vi "observacao.vi"() -> ()   [LabVIEW 2012] (continued)
                  frame True {
                    w2978 = u16 4 items=["ZERO", "AH", "DEC", "TUBO", "CUP"] ("Controlador")
                    n2288 = call "Monta Comando.vi"("Comando"="SUBIR", "Dispositivo"="PARAVENTO" ("Comando"), "Controlador"=w2978) -> ()  [unwired: 4 in, 3 out]
                  }
                }
              }
              event "BtParavDown": Value Change {
                n2289 = event-data() -> ("NewVal"=w2979:bool)  [unwired: 1 in, 5 out]
                n2290 = case shown="True" w2979 {
                  frame False {
                  }
                  frame True {
                    w2982 = u16 4 items=["ZERO", "AH", "DEC", "TUBO", "CUP"] ("Controlador")
                    n2291 = call "Monta Comando.vi"("Comando"="DESCER", "Dispositivo"="PARAVENTO" ("Comando"), "Controlador"=w2982) -> ()  [unwired: 4 in, 3 out]
                  }
                }
              }
              event "BtParavStop": Value Change {
                n2292 = event-data() -> ("NewVal"=w2983:bool)  [unwired: 1 in, 5 out]
                n2293 = case shown="True" w2983 {
                  frame False {
                  }
                  frame True {
                    w2986 = u16 4 items=["ZERO", "AH", "DEC", "TUBO", "CUP"] ("Controlador")
                    n2294 = call "Monta Comando.vi"("Comando"="PARAR", "Dispositivo"="PARAVENTO" ("Comando"), "Controlador"=w2986) -> ()  [unwired: 4 in, 3 out]
                  }
                }
              }
            }
            n2295 = global read "Global_Telescopio.vi" "PosCUP"() -> (w2830:i16)
            n2296 = local read "RefreshShutterState"() -> (w2831:bool)
            n2297 = call "Bit Status CUP.vi"("NomeStatus"=w2833) -> ("StatBit"=w2832:bool)
            "LedShutter" <- w2832
            n2298 = case shown="\"Stopping\"" w2838 {
              tunnel: w2834 -> [_ w2908 w2915 w2918]
              tunnel: w2835 -> [_ _ _ _]
              frame "", Default {
              }
              frame "Not Ready" {
                n2299 = case shown="False" w2908 {
                  frame False {
                    w2914 = u16 4 items=["ZERO", "AH", "DEC", "TUBO", "CUP"] ("Controlador")
                    n2300 = local read "DestCUP"() -> (w2910:i16)
                    n2301 = local write "StatDome"("Moving" ("Status")) -> ()
                    n2302 = Number To Decimal String(number=w2910) -> (decimal integer string=w2911:string)  [unwired: 1 in]
                    n2303 = call "Monta Comando.vi"("Set Point"=w2911, "Comando"="MOVER", "Dispositivo"="DOMO" ("Comando"), "Controlador"=w2914) -> ()  [unwired: 3 in, 3 out]
                  }
                  frame True {
                  }
                }
              }
              frame "Stopping" {
                n2304 = case shown="False" w2915 {
                  frame False {
                    # "Reabilita Abas"
                    n2305 = property on="Setup, Pointing & Guiding" class="TabCtl (strict)"("Page Selector Visible"=TRUE) -> ()  [unwired: 2 in, 2 out]
                    n2306 = local write "StatDome"("Stopped" ("Status")) -> ()
                  }
                  frame True {
                  }
                }
              }
              frame "Moving" {
                n2307 = case shown="False" w2918 {
                  frame False {
                    # "Reabilita Abas"
                    n2308 = property on="Setup, Pointing & Guiding" class="TabCtl (strict)"("Page Selector Visible"=TRUE) -> ()  [unwired: 2 in, 2 out]
                    n2309 = local write "StatDome"("Stopped" ("Status")) -> ()
                  }
                  frame True {
                  }
                }
              }
            }
            n2310 = case shown="\"Busy to Close\"" w2836 {
              tunnel: w2835 -> [_ _ _ _]
              tunnel: w2834 -> [_ w2891 w2897 _]
              frame "", Default {
              }
              frame "Busy to Open" {
                n2311 = case shown="False" w2891 {
                  frame False {
                    w2895 = u16 4 items=["ZERO", "AH", "DEC", "TUBO", "CUP"] ("Controlador")
                    n2312 = call "TickTimeout.vi"() -> ("msTick"=w2892:u32)  [unwired: 2 in, 2 out]
                    n2313 = local write "TimeoutTrap"(w2892) -> ()
                    n2314 = local write "StatShutter"("Moving" ("Status")) -> ()
                    n2315 = call "Monta Comando.vi"("Comando"="ABRIR", "Dispositivo"="TRAPEIRA" ("Comando"), "Controlador"=w2895) -> ()  [unwired: 4 in, 3 out]
                  }
                  frame True {
                  }
                }
              }
              frame "Busy to Close" {
                n2316 = case shown="False" w2897 {
                  frame False {
                    w2901 = u16 4 items=["ZERO", "AH", "DEC", "TUBO", "CUP"] ("Controlador")
                    n2317 = call "TickTimeout.vi"() -> ("msTick"=w2898:u32)  [unwired: 2 in, 2 out]
                    n2318 = local write "TimeoutTrap"(w2898) -> ()
                    n2319 = local write "StatShutter"("Moving" ("Status")) -> ()
                    n2320 = call "Monta Comando.vi"("Comando"="FECHAR", "Dispositivo"="TRAPEIRA" ("Comando"), "Controlador"=w2901) -> ()  [unwired: 4 in, 3 out]
                  }
                  frame True {
                  }
                }
              }
              frame "Moving" {
                n2321 = local read "TimeoutTrap"() -> (w2903:u32)
                n2322 = call "TickTimeout.vi"("msInicial"=w2903, "msTimeout"=u32 12000) -> ("Timeout"=w2904:bool)  [unwired: 2 out]
                n2323 = case shown="False" w2904 {
                  selector: w2904 -> [w2907 _]
                  frame False {
                    n2324 = Not(x=w2907) -> (.not. x?=w2906:bool)
                    n2325 = local write "RefreshShutterState"(w2906) -> ()
                  }
                  frame True {
                  }
                }
              }
            }
            n2326 = case shown="True" w2831 {
              selector: w2831 -> [_ w2886]
              tunnel: w2832 -> [_ w2887]
              frame False {
              }
              frame True {
                n2327 = Not(x=w2886) -> (.not. x?=→"RefreshShutterState":bool)
                n2328 = Select(t="Opened" ("Status"), s=w2887, f="Closed" ("Status")) -> (s? t:f=w2888:string)
                n2329 = local write "StatShutter"(w2888) -> ()
              }
            }
            n2330 = Divide(x=w2830, y=w2826) -> (x/y=w2841:dbl)
            n2331 = To Word Integer(number=w2841) -> (16bit integer=→"PosCup":i16)
            n2332 = local read "Flag-ShutClose"() -> (w2824:bool)
            n2333 = local read "Flag-ShutOpen"() -> (w2823:bool)
            n2334 = Or(x=w2824, y=w2823) -> (x .or. y?=w2822:bool)
            n2335 = case shown="True" w2822 {
              frame False {
              }
              frame True {
                n2336 = local read "Cont-ShutOpen"() -> (w2863:timestamp)
                n2337 = Get Date/Time In Seconds() -> (seconds since 1Jan1904=w2864:timestamp)
                n2338 = Greater Or Equal?(x=w2864, y=w2863) -> (x >= y?=w2862:bool)
                n2339 = case shown="True" w2862 {
                  frame False {
                  }
                  frame True {
                    w2866 = FALSE ("Flag-ShutClose")
                    # "Reabilita todas Abas"
                    n2340 = local write "Flag-ShutClose"(w2866) -> ()
                    n2341 = local write "Flag-ShutOpen"(w2866) -> ()
                    n2342 = property on="Setup, Pointing & Guiding" class="TabCtl (strict)"("Page Selector Visible"=TRUE) -> ()  [unwired: 2 in, 2 out]
                  }
                }
              }
            }
            n2343 = event shown="[2] \"BtShutOpen\": Value Change" {
              selector: _ -> [_ _ _]
              dyn-events: _ -> [_ _ _]
              timeout: 10 -> [_ _ _]
              event Timeout {
                n2344 = event-data() -> ()  [unwired: 1 in, 2 out]
              }
              event "BtShutClose": Value Change {
                # "Desabilita todas Abas"
                n2345 = event-data() -> ("NewVal"=w2867:bool)  [unwired: 1 in, 4 out]
                n2346 = case shown="True" w2867 {
                  selector: w2867 -> [_ w2872]
                  frame False {
                  }
                  frame True {
                    n2347 = Get Date/Time In Seconds() -> (seconds since 1Jan1904=w2871:timestamp)
                    n2348 = Add(x=w2871, y=10.0) -> (x+y=w2869:timestamp)
                    n2349 = local write "Cont-ShutOpen"(w2869) -> ()
                    n2350 = property on="Setup, Pointing & Guiding" class="TabCtl (strict)"("Page Selector Visible"=FALSE) -> ()  [unwired: 2 in, 2 out]
                    "Flag-ShutClose" <- w2872
                  }
                }
              }
              event "BtShutOpen": Value Change {
                # "Desabilita todas Abas"
                n2351 = event-data() -> ("NewVal"=w2873:bool)  [unwired: 1 in, 4 out]
                n2352 = case shown="True" w2873 {
                  selector: w2873 -> [_ w2874]
                  frame False {
                  }
                  frame True {
                    n2353 = stacked-sequence {
                      tunnel: w2874 -> [w2879 _]
                      frame #0 {
                        n2354 = Get Date/Time In Seconds() -> (seconds since 1Jan1904=w2878:timestamp)
                        n2355 = Add(x=w2878, y=10.0) -> (x+y=→"Cont-ShutOpen":timestamp)
                        n2356 = property on="Setup, Pointing & Guiding" class="TabCtl (strict)"("Page Selector Visible"=FALSE) -> ()  [unwired: 2 in, 2 out]
                        "Flag-ShutOpen" <- w2879
                      }
                      frame #1 {
                        # "Escreve no LOG o estado do shutter"
                        # "Timer para escrever no log\ne enviar comando:\nCUP TRAPEIRA PARAR"
                        n2357 = Tick Count (ms)() -> (millisecond timer value=w2880:u32)
                        n2358 = local write "sendCommandShutter"(TRUE ("writeShutterLog")) -> ()
                        n2359 = local write "timeStatShutterAlert"(w2880) -> ()
                        n2360 = local write "shutterTimeOld"(w2880) -> ()
                        n2361 = call "Log_Shutter.vi"("command"=" ", "domeState"="OPENED " ("command"), "pathLogDomeFile"="C:\\TCS\\LOG\\SHUTTER\\SHUTTER.TXT" ("pathLogFocoString")) -> ()  [unwired: 6 in]
                      }
                    }
                  }
                }
              }
            }
            n2362 = event shown="[3] \"CW\": Mouse Down" {
              selector: _ -> [_ _ _ _ _]
              dyn-events: _ -> [_ _ _ _ _]
              timeout: 100 -> [_ _ _ _ _]
              event Timeout {
                n2363 = event-data() -> ()  [unwired: 1 in, 2 out]
              }
              event "CCW": Mouse Down {
                w2842 = "GIRAR_CCW" ("Comando")
                w2843 = u16 4 items=["ZERO", "AH", "DEC", "TUBO", "CUP"] ("Controlador")
                # "Envia o comando GIRAR"
                n2364 = event-data() -> ()  [unwired: 1 in, 7 out]
                n2365 = local write "Command"(w2842) -> ()
                n2366 = call "Monta Comando.vi"("Comando"=w2842, "Dispositivo"="DOMO" ("Comando"), "Controlador"=w2843) -> ()  [unwired: 4 in, 3 out]
              }
              event "CCW": Mouse Up {
                n2367 = event-data() -> ()  [unwired: 1 in, 7 out]
                n2368 = stacked-sequence {
                  frame #0 {
                    w2845 = "PARAR" ("Comando")
                    w2846 = u16 4 items=["ZERO", "AH", "DEC", "TUBO", "CUP"] ("Controlador")
                    # "Envia o comando PARAR"
                    n2369 = local write "Command"(w2845) -> ()
                    n2370 = call "Monta Comando.vi"("Comando"=w2845, "Dispositivo"="DOMO" ("Comando"), "Controlador"=w2846) -> ()  [unwired: 4 in, 3 out]
                  }
                  frame #1 {
                    n2371 = Wait (ms)(milliseconds to wait=u32 100) -> ()  [unwired: 1 out]
                  }
                  frame #2 {
                    w2849 = "PARAR" ("Comando")
                    w2850 = u16 4 items=["ZERO", "AH", "DEC", "TUBO", "CUP"] ("Controlador")
                    # "Envia o comando PARAR"
                    n2372 = local write "Command"(w2849) -> ()
                    n2373 = call "Monta Comando.vi"("Comando"=w2849, "Dispositivo"="DOMO" ("Comando"), "Controlador"=w2850) -> ()  [unwired: 4 in, 3 out]
                  }
                }
              }
              event "CW": Mouse Down {
                w2852 = "GIRAR_CW" ("Comando")
                w2853 = u16 4 items=["ZERO", "AH", "DEC", "TUBO", "CUP"] ("Controlador")
                # "Envia o comando GIRAR"
                n2374 = event-data() -> ()  [unwired: 1 in, 7 out]
                n2375 = local write "Command"(w2852) -> ()
                n2376 = call "Monta Comando.vi"("Comando"=w2852, "Dispositivo"="DOMO" ("Comando"), "Controlador"=w2853) -> ()  [unwired: 4 in, 3 out]
              }
              event "CW": Mouse Up {
                n2377 = event-data() -> ()  [unwired: 1 in, 7 out]
                n2378 = stacked-sequence {
                  frame #0 {
                    w2855 = "PARAR" ("Comando")
                    w2856 = u16 4 items=["ZERO", "AH", "DEC", "TUBO", "CUP"] ("Controlador")
                    # "Envia o comando PARAR"
                    n2379 = local write "Command"(w2855) -> ()
                    n2380 = call "Monta Comando.vi"("Comando"=w2855, "Dispositivo"="DOMO" ("Comando"), "Controlador"=w2856) -> ()  [unwired: 4 in, 3 out]
                  }
                  frame #1 {
                    n2381 = Wait (ms)(milliseconds to wait=u32 100) -> ()  [unwired: 1 out]
                  }
                  frame #2 {
                    w2859 = "PARAR" ("Comando")
                    w2860 = u16 4 items=["ZERO", "AH", "DEC", "TUBO", "CUP"] ("Controlador")
                    # "Envia o comando PARAR"
                    n2382 = local write "Command"(w2859) -> ()
                    n2383 = call "Monta Comando.vi"("Comando"=w2859, "Dispositivo"="DOMO" ("Comando"), "Controlador"=w2860) -> ()  [unwired: 4 in, 3 out]
                  }
                }
              }
            }
            "Command" <- "" ("Command")
          }
          frame "UTILS " {
            n2384 = stacked-sequence {
              frame #0 {
                # "Acionamento das Abas do\nEspelho\n\nComandos sempre precedidos\nde ESPAÇO\n\nTUBO TAMPAS ESCREVER = 80 80\n\nLigar power geral       08 08\nDesligar power geral  08 00\nLigar System              10 10\nDesligar System         10 00\nPassar para Remoto  20 20\nPassar para Local      20 00\nSel. device central     40 40\nSel. device bowl         40 00\nAction open                80 80\nAction close                80 00"
                n2385 = event shown="[1] \"MODE\": Value Change" {
                  selector: _ -> [_ _ _]
                  dyn-events: _ -> [_ _ _]
                  timeout: 10 -> [_ _ _]
                  event Timeout {
                    n2386 = event-data() -> ()  [unwired: 1 in, 2 out]
                  }
                  event "MODE": Value Change {
                    n2387 = event-data() -> ("NewVal"=w3001:bool)  [unwired: 1 in, 5 out]
                    "LED MODE" <- w3001
                    n2388 = case shown="False" w3001 {
                      frame False {
                        w3006 = u16 3 items=["ZERO", "AH", "DEC", "TUBO", "CUP"] ("Controlador")
                        # "DESABILITA"
                        # "APENAS PASSANDO COMANDO PARA MANETE"
                        # "MODE E GERAL = 0"
                        # "MODE HADSET"
                        n2389 = call "Monta Comando.vi"("Set Point"=" F8 90", "Comando"="ESCREVER", "Dispositivo"="TAMPAS" ("Comando"), "Controlador"=w3006) -> ()  [unwired: 3 in, 3 out]
                        n2390 = property on="ACTION" class="Bool (strict)"("Disabled"=u8 2) -> ()  [unwired: 2 in, 2 out]
                      }
                      frame True {
                        w3011 = u16 3 items=["ZERO", "AH", "DEC", "TUBO", "CUP"] ("Controlador")
                        # "HABILITA"
                        # "APENAS PASSANDO COMOANDO PARA TCSPD"
                        # "MODE E GERAL = 1"
                        # "MODE TCSPD"
                        n2391 = call "Monta Comando.vi"("Set Point"=" 48 48", "Comando"="ESCREVER", "Dispositivo"="TAMPAS" ("Comando"), "Controlador"=w3011) -> ()  [unwired: 3 in, 3 out]
                        n2392 = property on="ACTION" class="Bool (strict)"("Disabled"=u8 0) -> ()  [unwired: 2 in, 2 out]
                      }
                    }
                  }
                  event "ACTION": Value Change {
                    n2393 = event-data() -> ("NewVal"=w3012:bool)  [unwired: 1 in, 5 out]
                    n2394 = case shown="False" w3012 {
                      frame False {
                        # "FECHAR"
                        n2395 = local write "ESTADO FECHAR"("INICIO" ("ESTADO ABRIR")) -> ()
                        n2396 = local write "ESTADO ABRIR"("REPOUSO" ("ESTADO ABRIR")) -> ()
                      }
                      frame True {
                        # "ABRIR"
                        n2397 = local write "ESTADO FECHAR"("REPOUSO" ("ESTADO ABRIR")) -> ()
                        n2398 = local write "ESTADO ABRIR"("INICIO" ("ESTADO ABRIR")) -> ()
                      }
                    }
                  }
                }
                n2399 = Tick Count (ms)() -> (millisecond timer value=w2992:u32)
                n2400 = Greater Or Equal?(x=w2992, y="TIMER TICK") -> (x >= y?=w2988:bool)
                n2401 = And(x=w2988, y=FALSE) -> (x .and. y?=w2989:bool)
                n2402 = case shown="True" w2989 {
                  frame False {
                  }
                  frame True {
                    w3025 = u16 3 items=["ZERO", "AH", "DEC", "TUBO", "CUP", "CASS", "COUDE"] ("Controlador")
                    # "2 SEGUNDOS"
                    n2403 = Tick Count (ms)() -> (millisecond timer value=w3022:u32)
                    n2404 = Add(x=w3022, y=u32 10000) -> (x+y=w3020:u32)
                    n2405 = call "Status_das_Tampas.vi"("Controlador"=w3025, "DISPOSITIVO"="TAMPAS", "Comando"="LER") -> ("Fechado/Aberto"=w3019:bool, "Dispositivo Bacia/Centar"=w3018:bool)  [unwired: 6 in, 5 out]
                    n2406 = local write "TIMER TICK"(w3020) -> ()
                    n2407 = Not(x=w3019) -> (.not. x?=w3017:bool)
                    n2408 = And(x=w3017, y=w3018) -> ()  [unwired: 1 out]
                  }
                }
                n2409 = event shown="[4] \"FLAT-FIELD\": Value Change" {
                  selector: _ -> [_ _ _ _ _ _]
                  dyn-events: _ -> [_ _ _ _ _ _]
                  timeout: 10 -> [_ _ _ _ _ _]
                  event Timeout {
                    n2410 = event-data() -> ()  [unwired: 1 in, 2 out]
                  }
                  event "BtUtilPark": Value Change {
                    n2411 = event-data() -> ("NewVal"=w3026:bool)  [unwired: 1 in, 5 out]
                    n2412 = case shown="True" w3026 {
                      frame False {
                      }
                      frame True {
                        w3029 = u16 4 items=["ZERO", "AH", "DEC", "TUBO", "CUP"] ("Controlador")
                        w3030 = FALSE ("MOUNT")
                        w3033 = 0 ("M_AH")
                        w3034 = u8 2 ("Disabled")
                        w3031 = FALSE ("Page Selector Visible")
                        w3038 = 1 ("M_AH")
                        # "Carrega \nParâmetros \nda Configuração"
                        # "Seta Máq GO"
                        # "Desabilita todas Abas"
                        # "DESABILITA TODOS"
                        n2413 = local write "DOME"(w3031) -> ()
                        n2414 = property on="Setup, Pointing & Guiding" class="TabCtl (strict)"("Page Selector Visible"=w3031) -> ()  [unwired: 2 in, 2 out]
                        n2415 = local write "statAH"(w3033) -> ()
                        n2416 = local write "statCUP"(w3033) -> ()
                        n2417 = local write "statDEC"(w3033) -> ()
                        n2418 = local write "M_DEC"(w3038) -> ()
                        n2419 = local write "M_AH"(w3038) -> ()
                        n2420 = local write "M_CUP"(w3038) -> ()
                        n2421 = global read "Global_Telescopio.vi" "DestDEC"() -> (w3036:dbl)
                        n2422 = global read "Global_Telescopio.vi" "DestCUP"() -> (w3035:i32)
                        n2423 = global read "Global_Telescopio.vi" "DestAH"() -> (w3037:dbl)
                        n2424 = property on="BtUtilPark" class="Bool (strict)"("Disabled"=w3034) -> ()  [unwired: 2 in, 2 out]
                        n2425 = property on="ECASS" class="Bool (strict)"("Disabled"=w3034) -> ()  [unwired: 2 in, 2 out]
                        n2426 = local write "DestAH"(w3037) -> ()
                        n2427 = local write "DestCUP"(w3035) -> ()
                        n2428 = local write "DestDEC"(w3036) -> ()
                        n2429 = global write "Global_Telescopio.vi" "Parking"(TRUE ("Page Selector Visible")) -> ()
                        n2430 = property on="BtUtilZenith" class="Bool (strict)"("Disabled"=w3034) -> ()  [unwired: 2 in, 2 out]
                        n2431 = property on="FLAT-FIELD" class="Bool (strict)"("Disabled"=w3034) -> ()  [unwired: 2 in, 2 out]
                        n2432 = call "Monta Comando.vi"("Comando"="LIGAR", "Dispositivo"="LAMP_CAM" ("Comando"), "Controlador"=w3029) -> ()  [unwired: 4 in, 3 out]
                        n2433 = property on="PROTEÇÃO" class="Bool (strict)"("Disabled"=w3034) -> ()  [unwired: 2 in, 2 out]
                        n2434 = local write "MOUNT"(w3030) -> ()
                        n2435 = local write "GUIDER"(w3030) -> ()
                      }
                    }
                  }
                  event "BtUtilZenith": Value Change {
                    n2436 = event-data() -> ("NewVal"=w3039:bool)  [unwired: 1 in, 5 out]
                    n2437 = case shown="True" w3039 {
                      frame False {
                      }
                      frame True {
                        w3042 = u16 4 items=["ZERO", "AH", "DEC", "TUBO", "CUP"] ("Controlador")
                        w3043 = FALSE ("MOUNT")
                        w3046 = 0 ("M_AH")
                        w3047 = u8 2 ("Disabled")
                        w3045 = FALSE ("Page Selector Visible")
                        w3051 = 1 ("M_AH")
                        # "Seta Máq GO"
                        # "Desabilita todas Abas"
                        # "DESABILITA TODOS"
                        n2438 = local write "M_DEC"(w3051) -> ()
                        n2439 = local write "M_AH"(w3051) -> ()
                        n2440 = local write "M_CUP"(w3051) -> ()
                        n2441 = local write "DOME"(w3045) -> ()
                        n2442 = property on="Setup, Pointing & Guiding" class="TabCtl (strict)"("Page Selector Visible"=w3045) -> ()  [unwired: 2 in, 2 out]
                        n2443 = local write "statAH"(w3046) -> ()
                        n2444 = local write "statCUP"(w3046) -> ()
                        n2445 = local write "statDEC"(w3046) -> ()
                        n2446 = global read "Global_Telescopio.vi" "Telescopio"() -> (w3044:bool)
                        n2447 = property on="BtUtilPark" class="Bool (strict)"("Disabled"=w3047) -> ()  [unwired: 2 in, 2 out]
                        n2448 = property on="ECASS" class="Bool (strict)"("Disabled"=w3047) -> ()  [unwired: 2 in, 2 out]
                        n2449 = case shown="False" w3044 {
                          tunnel: [0.0 ("DestAH") 0.0 ("DestAH")] -> w3050
                          tunnel: [-0.3933 ("DestDEC") -0.3933 ("DestDEC")] -> w3049
                          tunnel: [i16 98 ("DestCUP") i16 80 ("DestCUP")] -> w3048
                          frame False {
                          }
                          frame True {
                          }
                        }
                        n2450 = property on="BtUtilZenith" class="Bool (strict)"("Disabled"=w3047) -> ()  [unwired: 2 in, 2 out]
                        n2451 = property on="FLAT-FIELD" class="Bool (strict)"("Disabled"=w3047) -> ()  [unwired: 2 in, 2 out]
                        n2452 = call "Monta Comando.vi"("Comando"="LIGAR", "Dispositivo"="LAMP_CAM" ("Comando"), "Controlador"=w3042) -> ()  [unwired: 4 in, 3 out]
                        n2453 = local write "DestAH"(w3050) -> ()
                        n2454 = local write "DestCUP"(w3048) -> ()
                        n2455 = local write "DestDEC"(w3049) -> ()
                        n2456 = property on="PROTEÇÃO" class="Bool (strict)"("Disabled"=w3047) -> ()  [unwired: 2 in, 2 out]
                        n2457 = local write "MOUNT"(w3043) -> ()
                        n2458 = local write "GUIDER"(w3043) -> ()
                      }
                    }
                  }
                  event "ECASS": Value Change {
                    n2459 = event-data() -> ("NewVal"=w3058:bool)  [unwired: 1 in, 5 out]
                    n2460 = case shown="True" w3058 {
                      frame False {
                      }
                      frame True {
                        w3061 = u16 4 items=["ZERO", "AH", "DEC", "TUBO", "CUP"] ("Controlador")
                        w3062 = FALSE ("MOUNT")
                        w3065 = 0 ("M_AH")
                        w3066 = u8 2 ("Disabled")
                        w3064 = FALSE ("Page Selector Visible")
                        w3070 = 1 ("M_AH")
                        # "Seta Máq GO"
                        # "Desabilita todas Abas"
                        # "DESABILITA TODOS"
                        n2461 = local write "M_DEC"(w3070) -> ()
                        n2462 = local write "M_AH"(w3070) -> ()
                        n2463 = local write "M_CUP"(w3070) -> ()
                        n2464 = local write "DOME"(w3064) -> ()
                        n2465 = property on="Setup, Pointing & Guiding" class="TabCtl (strict)"("Page Selector Visible"=w3064) -> ()  [unwired: 2 in, 2 out]
                        n2466 = local write "statAH"(w3065) -> ()
                        n2467 = local write "statCUP"(w3065) -> ()
                        n2468 = local write "statDEC"(w3065) -> ()
                        n2469 = global read "Global_Telescopio.vi" "Telescopio"() -> (w3063:bool)
                        n2470 = property on="BtUtilPark" class="Bool (strict)"("Disabled"=w3066) -> ()  [unwired: 2 in, 2 out]
                        n2471 = property on="ECASS" class="Bool (strict)"("Disabled"=w3066) -> ()  [unwired: 2 in, 2 out]
                        n2472 = case shown="False" w3063 {
                          tunnel: [0.0 ("DestAH") 0.0 ("DestAH")] -> w3069
                          tunnel: [0.4 ("DestDEC") 0.4 ("DestDEC")] -> w3068
                          tunnel: [i16 98 ("DestCUP") i16 80 ("DestCUP")] -> w3067
                          frame False {
                          }
                          frame True {
                          }
                        }
                        n2473 = property on="BtUtilZenith" class="Bool (strict)"("Disabled"=w3066) -> ()  [unwired: 2 in, 2 out]
                        n2474 = property on="FLAT-FIELD" class="Bool (strict)"("Disabled"=w3066) -> ()  [unwired: 2 in, 2 out]
                        n2475 = local write "DestAH"(w3069) -> ()
                        n2476 = local write "DestCUP"(w3067) -> ()
                        n2477 = local write "DestDEC"(w3068) -> ()
                        n2478 = call "Monta Comando.vi"("Comando"="LIGAR", "Dispositivo"="LAMP_CAM" ("Comando"), "Controlador"=w3061) -> ()  [unwired: 4 in, 3 out]
                        n2479 = property on="PROTEÇÃO" class="Bool (strict)"("Disabled"=w3066) -> ()  [unwired: 2 in, 2 out]
                        n2480 = local write "GUIDER"(w3062) -> ()
                        n2481 = local write "MOUNT"(w3062) -> ()
                      }
                    }
                  }
                  event "FLAT-FIELD": Value Change {
                    n2482 = event-data() -> ("NewVal"=w3077:bool)  [unwired: 1 in, 5 out]
                    n2483 = case shown="True" w3077 {
                      frame False {
                      }
                      frame True {
                        w3080 = u16 4 items=["ZERO", "AH", "DEC", "TUBO", "CUP"] ("Controlador")
                        w3081 = FALSE ("MOUNT")
                        w3083 = 0 ("M_AH")
                        w3085 = u8 2 ("Disabled")
                        w3084 = FALSE ("Page Selector Visible")
                        w3089 = 1 ("M_AH")
                        # "Seta Máq GO"
                        # "Desabilita todas Abas"
                        # "DESABILITA TODOS"
                        n2484 = local write "M_DEC"(w3089) -> ()
                        n2485 = local write "M_AH"(w3089) -> ()
                        n2486 = local write "M_CUP"(w3089) -> ()
                        n2487 = local write "DOME"(w3084) -> ()
                        n2488 = property on="Setup, Pointing & Guiding" class="TabCtl (strict)"("Page Selector Visible"=w3084) -> ()  [unwired: 2 in, 2 out]
                        n2489 = local write "statAH"(w3083) -> ()
                        n2490 = local write "statCUP"(w3083) -> ()
                        n2491 = local write "statDEC"(w3083) -> ()
                        n2492 = global read "Global_Telescopio.vi" "Telescopio"() -> (w3082:bool)
                        n2493 = property on="BtUtilPark" class="Bool (strict)"("Disabled"=w3085) -> ()  [unwired: 2 in, 2 out]
                        n2494 = property on="ECASS" class="Bool (strict)"("Disabled"=w3085) -> ()  [unwired: 2 in, 2 out]
                        n2495 = case shown="False" w3082 {
                          tunnel: [0.0715 ("DestAH") 0.31416 ("DestAH")] -> w3088
                          tunnel: [0.641 ("DestDEC") -0.39415 ("DestDEC")] -> w3087
                          tunnel: [i16 306 ("DestCUP") i16 133 ("DestCUP")] -> w3086
                          frame False {
                          }
                          frame True {
                          }
                        }
                        n2496 = property on="BtUtilZenith" class="Bool (strict)"("Disabled"=w3085) -> ()  [unwired: 2 in, 2 out]
                        n2497 = property on="FLAT-FIELD" class="Bool (strict)"("Disabled"=w3085) -> ()  [unwired: 2 in, 2 out]
                        n2498 = local write "DestAH"(w3088) -> ()
                        n2499 = local write "DestCUP"(w3086) -> ()
                        n2500 = local write "DestDEC"(w3087) -> ()
                        n2501 = call "Monta Comando.vi"("Comando"="LIGAR", "Dispositivo"="LAMP_CAM" ("Comando"), "Controlador"=w3080) -> ()  [unwired: 4 in, 3 out]
                        n2502 = property on="PROTEÇÃO" class="Bool (strict)"("Disabled"=w3085) -> ()  [unwired: 2 in, 2 out]
                        n2503 = local write "GUIDER"(w3081) -> ()
                        n2504 = local write "MOUNT"(w3081) -> ()
                      }
                    }
                  }
                  event "PROTEÇÃO": Value Change {
                    n2505 = event-data() -> ("NewVal"=w3096:bool)  [unwired: 1 in, 5 out]
                    n2506 = case shown="True" w3096 {
                      frame False {
                      }
                      frame True {
                        w3097 = FALSE ("MOUNT")
                        w3099 = 0 ("M_AH")
                        w3098 = FALSE ("Page Selector Visible")
                        w3101 = u8 2 ("Disabled")
                        # "Seta Máq GO"
                        # "Desabilita todas Abas"
                        # "DESABILITA TODOS"
                        n2507 = local write "DOME"(w3098) -> ()
                        n2508 = property on="Setup, Pointing & Guiding" class="TabCtl (strict)"("Page Selector Visible"=w3098) -> ()  [unwired: 2 in, 2 out]
                        n2509 = local write "statAH"(w3099) -> ()
                        n2510 = local write "statCUP"(w3099) -> ()
                        n2511 = local write "statDEC"(w3099) -> ()
                        n2512 = property on="BtUtilPark" class="Bool (strict)"("Disabled"=w3101) -> ()  [unwired: 2 in, 2 out]
                        n2513 = property on="ECASS" class="Bool (strict)"("Disabled"=w3101) -> ()  [unwired: 2 in, 2 out]
                        n2514 = property on="BtUtilZenith" class="Bool (strict)"("Disabled"=w3101) -> ()  [unwired: 2 in, 2 out]
                        n2515 = property on="FLAT-FIELD" class="Bool (strict)"("Disabled"=w3101) -> ()  [unwired: 2 in, 2 out]
                        n2516 = local write "M_PROT"(1 ("M_PROT")) -> ()
                        n2517 = local write "GUIDER"(w3097) -> ()
                        n2518 = local write "MOUNT"(w3097) -> ()
                        n2519 = property on="PROTEÇÃO" class="Bool (strict)"("Disabled"=w3101) -> ()  [unwired: 2 in, 2 out]
                      }
                    }
                  }
                }
                n2520 = case shown="True" "STOP" {
                  frame False {
                  }
                  frame True {
                    n2521 = stacked-sequence {
                      frame #0 {
                        w3103 = 0 ("estado")
                        # "Zera Máquina de Estado\nPelo Botão STOP"
                        n2522 = property on="Setup, Pointing & Guiding" class="TabCtl (strict)"("Page Selector Visible"=TRUE) -> ()  [unwired: 2 in, 2 out]
                        n2523 = call "Stop.vi"() -> ()  [unwired: 1 in, 1 out]
                        n2524 = local write "Flag Stop"(TRUE ("Flag Stop")) -> ()
                        n2525 = local write "M_AH"(w3103) -> ()
                        n2526 = local write "M_DEC"(w3103) -> ()
                        n2527 = local write "M_CUP"(w3103) -> ()
                        n2528 = local write "M_PROT"(w3103) -> ()
                      }
                      frame #1 {
                        w3105 = FALSE
                        w3106 = u8 0 ("Disabled")
                        # "DESLIGA TODOS"
                        # "HABILITA TODOS"
                        n2529 = local write "BtUtilZenith"(w3105) -> ()
                        n2530 = local write "BtUtilPark"(w3105) -> ()
                        n2531 = local write "FLAT-FIELD"(w3105) -> ()
                        n2532 = local write "PROTEÇÃO"(w3105) -> ()
                        n2533 = local write "ECASS"(w3105) -> ()
                        n2534 = property on="BtUtilPark" class="Bool (strict)"("Disabled"=w3106) -> ()  [unwired: 2 in, 2 out]
                        n2535 = property on="ECASS" class="Bool (strict)"("Disabled"=w3106) -> ()  [unwired: 2 in, 2 out]
                        n2536 = property on="BtUtilZenith" class="Bool (strict)"("Disabled"=w3106) -> ()  [unwired: 2 in, 2 out]
                        n2537 = property on="PROTEÇÃO" class="Bool (strict)"("Disabled"=w3106) -> ()  [unwired: 2 in, 2 out]
                        n2538 = property on="FLAT-FIELD" class="Bool (strict)"("Disabled"=w3106) -> ()  [unwired: 2 in, 2 out]
                      }
                    }
                  }
                }
                n2539 = Compound Arithmetic op=OR("BtUtilPark", "BtUtilZenith", "ECASS", "FLAT-FIELD", "PROTEÇÃO") -> (→"MOVING":bool)
              }
              frame #1 {
                # "MÁQUINAS DE ESTADOS DAS TAMPAS"
                n2540 = case shown="False" "Case Constant\n(See Context Help) 11" {
                  frame False {
                    # "ABRIR"
                    # "FECHAR"
                    n2541 = case shown="\"PIZZA\"" "ESTADO FECHAR" {
                      tunnel: [w3157 w3165 w3176 w3184 w3194 w3202 w3212 "REPOUSO" ("y")] -> w3111
                      frame "INICIO", Default {
                        w3162 = u16 3 items=["ZERO", "AH", "DEC", "TUBO", "CUP"] ("Controlador")
                        # "SELECIONA DISPOSITVO BACIA E\nMANDA FECHAR"
                        # "DISP=1 E PIZZA=1"
                        n2542 = call "Monta Comando.vi"("Set Point"=" A0 A0", "Comando"="ESCREVER", "Dispositivo"="TAMPAS" ("Comando"), "Controlador"=w3162) -> ("Resposta"=w3158:string)  [unwired: 3 in, 2 out]
                        n2543 = Not Equal?(x=w3158, y="TAMPAS OK") -> ()  [unwired: 1 out]
                        n2544 = Tick Count (ms)() -> (millisecond timer value=→"T1 2":u32)
                        n2545 = Select(t="REPOUSO" ("y"), s=FALSE, f="ESPERA 1" ("y")) -> (s? t:f=w3157:string)
                      }
                      frame "ESPERA 1" {
                        # "20 SEGUNDOS"
                        n2546 = local read "T1 2"() -> (w3170:u32)
                        n2547 = Tick Count (ms)() -> (millisecond timer value=w3168:u32)
                        n2548 = Add(x=w3170, y=u32 20000) -> (x+y=w3167:u32)
                        n2549 = Greater?(x=w3168, y=w3167) -> (0:w3164:bool)
                        n2550 = Select(t="PIZZA" ("y"), s=w3164, f="ESPERA 1" ("y")) -> (s? t:f=w3165:string)
                      }
                      frame "PIZZA" {
                        w3181 = u16 3 items=["ZERO", "AH", "DEC", "TUBO", "CUP"] ("Controlador")
                        # "SELECIONA DISP PIZZA\nE MANDA FECHAR"
                        # "PIZZA=1"
                        n2551 = call "Monta Comando.vi"("Set Point"=" 30 10", "Comando"="ESCREVER", "Dispositivo"="TAMPAS" ("Comando"), "Controlador"=w3181) -> ("Resposta"=w3175:string)  [unwired: 3 in, 2 out]
                        n2552 = Tick Count (ms)() -> (millisecond timer value=→"T2 2":u32)
                        n2553 = Not Equal?(x=w3175, y="TAMPAS OK") -> ()  [unwired: 1 out]
                        n2554 = Select(t="REPOUSO" ("y"), s=FALSE, f="PIZZA 2") -> (s? t:f=w3176:string)
                      }
                      frame "PIZZA 2" {
                        w3192 = u16 3 items=["ZERO", "AH", "DEC", "TUBO", "CUP"] ("Controlador")
                        n2555 = call "Monta Comando.vi"("Set Point"=" F8 90", "Comando"="ESCREVER", "Dispositivo"="TAMPAS" ("Comando"), "Controlador"=w3192) -> ("Resposta"=w3187:string)  [unwired: 3 in, 2 out]
                        n2556 = Tick Count (ms)() -> (millisecond timer value=→"T2 3":u32)
                        n2557 = Not Equal?(x=w3187, y="TAMPAS OK") -> ()  [unwired: 1 out]
                        n2558 = Select(t="REPOUSO" ("y"), s=FALSE, f="ESPERA 1A") -> (s? t:f=w3184:string)
                      }
                      frame "ESPERA 1A" {
                        # "2 SEGUNDOS"
                        n2559 = local read "T2 3"() -> (w3197:u32)
                        n2560 = Tick Count (ms)() -> (millisecond timer value=w3199:u32)
                        n2561 = Add(x=w3197, y=u32 2000) -> (x+y=w3200:u32)
                        n2562 = Greater?(x=w3199, y=w3200) -> (0:w3193:bool)
                        n2563 = Select(t="PIZZA 3" ("y"), s=w3193, f="ESPERA 1A" ("y")) -> (s? t:f=w3194:string)
                      }
                      frame "PIZZA 3" {
                        w3210 = u16 3 items=["ZERO", "AH", "DEC", "TUBO", "CUP"] ("Controlador")
                        # "PIZZA=3"
                        n2564 = call "Monta Comando.vi"("Set Point"=" 48 48", "Comando"="ESCREVER", "Dispositivo"="TAMPAS" ("Comando"), "Controlador"=w3210) -> ("Resposta"=w3205:string)  [unwired: 3 in, 2 out]
                        n2565 = Not Equal?(x=w3205, y="TAMPAS OK") -> ()  [unwired: 1 out]
                        n2566 = Select(t="REPOUSO" ("y"), s=FALSE, f="ESPERA 2" ("y")) -> (s? t:f=w3202:string)
                      }
                      frame "ESPERA 2" {
                        # "10 SEGUNDOS"
                        n2567 = local read "T2 2"() -> (w3216:u32)
                        n2568 = Tick Count (ms)() -> (millisecond timer value=w3214:u32)
                        n2569 = Add(x=w3216, y=u32 10000) -> (x+y=w3213:u32)
                        n2570 = Greater?(x=w3214, y=w3213) -> (0:w3211:bool)
                        n2571 = case shown="True" w3211 {
                          frame False {
                          }
                          frame True {
                            n2572 = local write "LED ACTION"(FALSE ("LED ACTION")) -> ()
                          }
                        }
                        n2573 = Select(t="REPOUSO" ("y"), s=w3211, f="ESPERA 2" ("y")) -> (s? t:f=w3212:string)
                      }
                      frame "REPOUSO" {
                      }
                    }
                    n2574 = local write "ESTADO FECHAR"(w3111) -> ()
                    n2575 = case shown="\"INICIO\", Default" "ESTADO ABRIR" {
                      tunnel: [w3116 w3125 w3136 w3143 "REPOUSO" ("y")] -> w3109
                      frame "INICIO", Default {
                        w3122 = u16 3 items=["ZERO", "AH", "DEC", "TUBO", "CUP"] ("Controlador")
                        # "SELECIONA DISPOSITVO PIZZA E\nMANDA ABRIR"
                        # "DISP=0 E PIZZA=0"
                        n2576 = call "Monta Comando.vi"("Set Point"=" 30 00", "Comando"="ESCREVER", "Dispositivo"="TAMPAS" ("Comando"), "Controlador"=w3122) -> ("Resposta"=w3117:string)  [unwired: 3 in, 2 out]
                        n2577 = Not Equal?(x=w3117, y="TAMPAS OK") -> ()  [unwired: 1 out]
                        n2578 = Tick Count (ms)() -> (millisecond timer value=→"T1":u32)
                        n2579 = Select(t="REPOUSO" ("y"), s=FALSE, f="ESPERA 1" ("y")) -> (s? t:f=w3116:string)
                      }
                      frame "ESPERA 1" {
                        # "10 SEGUNDOS"
                        n2580 = local read "T1"() -> (w3130:u32)
                        n2581 = Tick Count (ms)() -> (millisecond timer value=w3128:u32)
                        n2582 = Add(x=w3130, y=u32 10000) -> (x+y=w3127:u32)
                        n2583 = Greater?(x=w3128, y=w3127) -> (0:w3124:bool)
                        n2584 = Select(t="BACIA" ("y"), s=w3124, f="ESPERA 1" ("y")) -> (s? t:f=w3125:string)
                      }
                      frame "BACIA" {
                        w3141 = u16 3 items=["ZERO", "AH", "DEC", "TUBO", "CUP"] ("Controlador")
                        # "SELECIONA DISP BACIA\nE MANDA ABRIR"
                        # "BACIA=0"
                        n2585 = call "Monta Comando.vi"("Set Point"=" A0 20", "Comando"="ESCREVER", "Dispositivo"="TAMPAS" ("Comando"), "Controlador"=w3141) -> ("Resposta"=w3135:string)  [unwired: 3 in, 2 out]
                        n2586 = Tick Count (ms)() -> (millisecond timer value=→"T2":u32)
                        n2587 = Not Equal?(x=w3135, y="TAMPAS OK") -> ()  [unwired: 1 out]
                        n2588 = Select(t="REPOUSO" ("y"), s=FALSE, f="ESPERA 2") -> (s? t:f=w3136:string)
                      }
                      frame "ESPERA 2" {
                        # "25 SEGUNDOS"
                        n2589 = local read "T2"() -> (w3147:u32)
                        n2590 = Tick Count (ms)() -> (millisecond timer value=w3145:u32)
                        n2591 = Add(x=w3147, y=u32 25000) -> (x+y=w3144:u32)
                        n2592 = Greater?(x=w3145, y=w3144) -> (0:w3142:bool)
                        n2593 = case shown="True" w3142 {
                          frame False {
                          }
                          frame True {
                            n2594 = local write "LED ACTION"(TRUE ("LED ACTION")) -> ()
                          }
                        }
                        n2595 = Select(t="REPOUSO" ("y"), s=w3142, f="ESPERA 2" ("y")) -> (s? t:f=w3143:string)
                      }
                      frame "REPOUSO" {
                      }
                    }
                    n2596 = local write "ESTADO ABRIR"(w3109) -> ()
                  }
                  frame True {
                    # "NOVO"
                    # "ABRIR"
                    # "FECHAR"
                    n2597 = local read "ESTADO FECHAR"() -> (w3224:string)
                    n2598 = case shown="\"INICIO\", Default" w3224 {
                      tunnel: [w3289 w3297 w3308 w3316 w3324 "REPOUSO" ("y")] -> w3223
                      frame "INICIO", Default {
                        w3294 = u16 3 items=["ZERO", "AH", "DEC", "TUBO", "CUP"] ("Controlador")
                        # "SELECIONA DISPOSITVO BACIA E\nMANDA FECHAR"
                        n2599 = call "Monta Comando.vi"("Set Point"=" A0 A0", "Comando"="ESCREVER", "Dispositivo"="TAMPAS" ("Comando"), "Controlador"=w3294) -> ("Resposta"=w3290:string)  [unwired: 3 in, 2 out]
                        n2600 = Not Equal?(x=w3290, y="TAMPAS OK") -> ()  [unwired: 1 out]
                        n2601 = Tick Count (ms)() -> (millisecond timer value=→"TF1":u32)
                        n2602 = Select(t="REPOUSO" ("y"), s=FALSE, f="ESPERA1" ("y")) -> (s? t:f=w3289:string)
                      }
                      frame "ESPERA1" {
                        # "20 SEGUNDOS"
                        n2603 = local read "TF1"() -> (w3302:u32)
                        n2604 = Tick Count (ms)() -> (millisecond timer value=w3300:u32)
                        n2605 = Add(x=w3302, y=u32 20000) -> (x+y=w3299:u32)
                        n2606 = Greater?(x=w3300, y=w3299) -> (0:w3296:bool)
                        n2607 = Select(t="PIZZA" ("y"), s=w3296, f="ESPERA1" ("y")) -> (s? t:f=w3297:string)
                      }
                      frame "PIZZA" {
                        w3313 = u16 3 items=["ZERO", "AH", "DEC", "TUBO", "CUP"] ("Controlador")
                        # "PASSA PARA MODO\nHANDSET E PIZZA FECHA"
                        n2608 = call "Monta Comando.vi"("Set Point"=" 48 00", "Comando"="ESCREVER", "Dispositivo"="TAMPAS" ("Comando"), "Controlador"=w3313) -> ("Resposta"=w3307:string)  [unwired: 3 in, 2 out]
                        n2609 = Tick Count (ms)() -> (millisecond timer value=→"TF2":u32)
                        n2610 = Not Equal?(x=w3307, y="TAMPAS OK") -> ()  [unwired: 1 out]
                        n2611 = Select(t="REPOUSO" ("y"), s=FALSE, f="ESPERA2") -> (s? t:f=w3308:string)
                      }
                      frame "ESPERA2" {
                        # "10 SEGUNDOS"
                        n2612 = local read "TF2"() -> (w3314:u32)
                        n2613 = Tick Count (ms)() -> (millisecond timer value=w3320:u32)
                        n2614 = Add(x=w3314, y=u32 10000) -> (x+y=w3321:u32)
                        n2615 = Greater?(x=w3320, y=w3321) -> (0:w3315:bool)
                        n2616 = Select(t="PIZZA3" ("y"), s=w3315, f="ESPERA2" ("y")) -> (s? t:f=w3316:string)
                      }
                      frame "PIZZA3" {
                        w3332 = u16 3 items=["ZERO", "AH", "DEC", "TUBO", "CUP"] ("Controlador")
                        n2617 = case shown="True" "Case Constant\n(See Context Help) 12" {
                          frame False {
                          }
                          frame True {
                            n2618 = local write "LED ACTION"(FALSE ("LED ACTION")) -> ()
                          }
                        }
                        n2619 = call "Monta Comando.vi"("Set Point"=" 48 48", "Comando"="ESCREVER", "Dispositivo"="TAMPAS" ("Comando"), "Controlador"=w3332) -> ("Resposta"=w3327:string)  [unwired: 3 in, 2 out]
                        n2620 = Not Equal?(x=w3327, y="TAMPAS OK") -> ()  [unwired: 1 out]
                        n2621 = Select(t="REPOUSO" ("y"), s=FALSE, f="REPOUSO" ("y")) -> (s? t:f=w3324:string)
                      }
                      frame "REPOUSO" {
                      }
                    }
                    n2622 = local write "ESTADO FECHAR"(w3223) -> ()
                    n2623 = local read "ESTADO ABRIR"() -> (w3222:string)
                    n2624 = case shown="\"INICIO\", Default" w3222 {
                      tunnel: [w3229 w3237 w3245 w3255 w3264 w3277 "REPOUSO" ("y")] -> w3221
                      frame "INICIO", Default {
                        w3235 = u16 3 items=["ZERO", "AH", "DEC", "TUBO", "CUP"] ("Controlador")
                        # "PASSA PARA MODO HANDSET"
                        n2625 = call "Monta Comando.vi"("Set Point"=" F8 00", "Comando"="ESCREVER", "Dispositivo"="TAMPAS" ("Comando"), "Controlador"=w3235) -> ("Resposta"=w3230:string)  [unwired: 3 in, 2 out]
                        n2626 = Not Equal?(x=w3230, y="TAMPAS OK") -> ()  [unwired: 1 out]
                        n2627 = Tick Count (ms)() -> (millisecond timer value=→"TA1":u32)
                        n2628 = Select(t="REPOUSO" ("y"), s=FALSE, f="ESPERA1" ("y")) -> (s? t:f=w3229:string)
                      }
                      frame "ESPERA1" {
                        # "1 SEGUNDO"
                        n2629 = local read "TA1"() -> (w3236:u32)
                        n2630 = Tick Count (ms)() -> (millisecond timer value=w3242:u32)
                        n2631 = Add(x=w3236, y=u32 1000) -> (x+y=w3241:u32)
                        n2632 = Greater?(x=w3242, y=w3241) -> (0:w3239:bool)
                        n2633 = Select(t="ABREPIZZA" ("y"), s=w3239, f="ESPERA1" ("y")) -> (s? t:f=w3237:string)
                      }
                      frame "ABREPIZZA" {
                        w3254 = u16 3 items=["ZERO", "AH", "DEC", "TUBO", "CUP"] ("Controlador")
                        # "MANDA PIZZA ABRIR"
                        n2634 = call "Monta Comando.vi"("Set Point"=" 48 48", "Comando"="ESCREVER", "Dispositivo"="TAMPAS" ("Comando"), "Controlador"=w3254) -> ("Resposta"=w3249:string)  [unwired: 3 in, 2 out]
                        n2635 = Not Equal?(x=w3249, y="TAMPAS OK") -> ()  [unwired: 1 out]
                        n2636 = Tick Count (ms)() -> (millisecond timer value=→"TA2":u32)
                        n2637 = Select(t="ABREPIZZA" ("y"), s=FALSE, f="ESPERA2" ("y")) -> (s? t:f=w3245:string)
                      }
                      frame "ESPERA2" {
                        # "10 SEGUNDOS"
                        n2638 = local read "TA2"() -> (w3256:u32)
                        n2639 = Tick Count (ms)() -> (millisecond timer value=w3261:u32)
                        n2640 = Add(x=w3256, y=u32 10000) -> (x+y=w3260:u32)
                        n2641 = Greater?(x=w3261, y=w3260) -> (0:w3258:bool)
                        n2642 = Select(t="BACIAABRINDO" ("y"), s=w3258, f="ESPERA2" ("y")) -> (s? t:f=w3255:string)
                      }
                      frame "BACIAABRINDO" {
                        w3273 = u16 3 items=["ZERO", "AH", "DEC", "TUBO", "CUP"] ("Controlador")
                        # "BACIA ABRINDO"
                        n2643 = call "Monta Comando.vi"("Set Point"=" A0 20", "Comando"="ESCREVER", "Dispositivo"="TAMPAS" ("Comando"), "Controlador"=w3273) -> ("Resposta"=w3268:string)  [unwired: 3 in, 2 out]
                        n2644 = Not Equal?(x=w3268, y="TAMPAS OK") -> ()  [unwired: 1 out]
                        n2645 = Tick Count (ms)() -> (millisecond timer value=→"TA3":u32)
                        n2646 = Select(t="BACIAABRINDO" ("y"), s=FALSE, f="ESPERA3" ("y")) -> (s? t:f=w3264:string)
                      }
                      frame "ESPERA3" {
                        # "25 SEGUNDOS"
                        n2647 = local read "TA3"() -> (w3275:u32)
                        n2648 = Tick Count (ms)() -> (millisecond timer value=w3280:u32)
                        n2649 = Add(x=w3275, y=u32 25000) -> (x+y=w3279:u32)
                        n2650 = Greater?(x=w3280, y=w3279) -> (0:w3274:bool)
                        n2651 = case shown="True" w3274 {
                          frame False {
                          }
                          frame True {
                            n2652 = local write "LED ACTION"(TRUE ("LED ACTION")) -> ()
                          }
                        }
                        n2653 = Select(t="REPOUSO" ("y"), s=w3274, f="ESPERA3" ("y")) -> (s? t:f=w3277:string)
                      }
                      frame "REPOUSO" {
                      }
                    }
                    n2654 = local write "ESTADO ABRIR"(w3221) -> ()
                  }
                }
              }
              frame #2 {
                # "MÁQUINA DE ESTADOS PROTEÇÃO"
                n2655 = case shown="3" "M_PROT" {
                  selector: "M_PROT" -> [w3338 _ _ _ _ _]
                  tunnel: [w3338 w3339 w3358 5 5 ("estadoCUP") 0 ("estadoCUP")] -> w3336
                  frame 0, Default {
                    # "Sem movimento"
                    n2656 = call "TickTimeout.vi"() -> ("msTick"=→"Timeout PROT":u32)  [unwired: 2 in, 2 out]
                  }
                  frame 1 {
                    w3342 = u16 3 items=["Alarme", "Atencao", "Erro", "Ocupado", "Protecao", "Embreagem", "Tracking", "Var. Track", "Rápido", "Ligeiro", "Médio", "Lento", "Em movimento", ""] ("NomeStatus")
                    w3341 = u16 3 items=["Alarme", "Atencao", "Erro", "Ocupado", "Protecao", "Embreagem", "Tracking", "Var. Track", "Rápido", "Ligeiro", "Médio", "Lento", "Em movimento", ""] ("NomeStatus")
                    # "Testa Ocupado"
                    n2657 = call "Bit Status DEC.vi"("NomeStatus"=w3341) -> ("StatBit"=w3343:bool)
                    n2658 = call "Bit Status AH.vi"("NomeStatus"=w3342) -> ("StatBit"=w3344:bool)
                    n2659 = Or(x=w3344, y=w3343) -> (x .or. y?=w3340:bool)
                    n2660 = case shown="False" w3340 {
                      tunnel: [2 w3355] -> w3339
                      frame False {
                        w3351 = u16 2 items=["ZERO", "AH", "DEC", "TUBO", "CUP"] ("Controlador")
                        w3346 = u16 1 items=["ZERO", "AH", "DEC", "TUBO", "CUP"] ("Controlador")
                        # "Comando para os controladores\nsaírem da Proteção"
                        n2661 = call "Monta Comando.vi"("Comando"="LIBERAR", "Dispositivo"="EIXO" ("Comando"), "Controlador"=w3346) -> ()  [unwired: 4 in, 3 out]
                        n2662 = call "Monta Comando.vi"("Comando"="LIBERAR", "Dispositivo"="EIXO" ("Comando"), "Controlador"=w3351) -> ()  [unwired: 4 in, 3 out]
                      }
                      frame True {
                        # "Busy"
                        n2663 = local read "Timeout PROT"() -> (w3354:u32)
                        n2664 = call "TickTimeout.vi"("msInicial"=w3354, "msTimeout"=u32 20000) -> ("Timeout"=w3352:bool)  [unwired: 2 out]
                        n2665 = case shown="False" w3352 {
                          tunnel: [1 3] -> w3355
                          frame False {
                          }
                          frame True {
                          }
                        }
                      }
                    }
                  }
                  frame 2 {
                    # "Cálculos rápidos"
                    # "Vem do Setup"
                    # "Aguarda Sair da proteção"
                    n2666 = global read "Global_Telescopio.vi" "Zenital angle GRAUS"() -> (w3361:dbl)
                    n2667 = global read "Global_Telescopio.vi" "Z_LIBERA_GRAUS"() -> (w3360:dbl)
                    n2668 = Less?(x=w3361, y=w3360) -> (x < y?=w3359:bool)
                    n2669 = case shown="True" w3359 {
                      tunnel: [2 ("estadoCUP") 4 ("estadoCUP")] -> w3358
                      frame False {
                      }
                      frame True {
                        # "stop"
                      }
                    }
                  }
                  frame 3 {
                    w3364 = "TENTE NOVAMENTE" ("SYSTEM MESSAGES")
                    # "Trata Timeout"
                    n2670 = call "TickTimeout.vi"() -> ("msTick"=w3365:u32)  [unwired: 2 in, 2 out]
                    n2671 = call "Monta_Mensagem.vi"("Mensagem"=w3364) -> ()  [unwired: 2 in]
                    n2672 = call "Salva_systems_messages.vi"("Mensagem"=w3364) -> ()  [unwired: 5 in]
                    n2673 = local write "Timeout PROT"(w3365) -> ()
                  }
                  frame 4 {
                    w3368 = u16 1 items=["ZERO", "AH", "DEC", "TUBO", "CUP"] ("Controlador")
                    w3373 = u16 2 items=["ZERO", "AH", "DEC", "TUBO", "CUP"] ("Controlador")
                    # "Para os motores"
                    n2674 = call "Monta Comando.vi"("Comando"="PARAR", "Dispositivo"="PROG", "Controlador"=w3368) -> ()  [unwired: 4 in, 3 out]
                    n2675 = call "Monta Comando.vi"("Comando"="PARAR", "Dispositivo"="PROG", "Controlador"=w3373) -> ()  [unwired: 4 in, 3 out]
                  }
                  frame 5 {
                    # "SAÍDA"
                  }
                }
                n2676 = local write "M_PROT"(w3336) -> ()
              }
              frame #3 {
                w3392 = u16 3 items=["Alarme", "Atencao", "Erro", "Ocupado", "TBD", "LCB", "Trapeira", "Paravento", "DomoRap", "DomoCW", "DomoCCW", "TBD", "Em movimento", "TBD"] ("NomeStatus")
                w3400 = u16 3 items=["Alarme", "Atencao", "Erro", "Ocupado", "Protecao", "Embreagem", "Tracking", "Var. Track", "Rápido", "Ligeiro", "Médio", "Lento", "Em movimento", ""] ("NomeStatus")
                w3401 = u16 3 items=["Alarme", "Atencao", "Erro", "Ocupado", "Protecao", "Embreagem", "Tracking", "Var. Track", "Rápido", "Ligeiro", "Médio", "Lento", "Em movimento", ""] ("NomeStatus")
                n2677 = global read "Global_Telescopio.vi" "LimiarRapMed"() -> (w3402:dbl)
                n2678 = global read "Global_Telescopio.vi" "PosAH"() -> (w3404:dbl)
                n2679 = global read "Global_Telescopio.vi" "ErroMaxEixo"() -> (w3399:dbl)
                n2680 = global read "Global_Telescopio.vi" "PosDEC"() -> (w3403:dbl)
                n2681 = call "Bit Status DEC.vi"("NomeStatus"=w3400) -> ("StatBit"=w3398:bool)
                n2682 = call "Bit Status AH.vi"("NomeStatus"=w3401) -> ("StatBit"=w3397:bool)
                n2683 = case shown="4" "M_DEC" {
                  selector: "M_DEC" -> [w3501 _ _ _ _ _ _ _ _]
                  tunnel: [w3501 w3507 w3534 w3559 w3582 w3606 0 w3623 w3628] -> w3381
                  tunnel: "DestDEC" -> [_ w3506 w3531 w3553 w3579 _ _ _ _]
                  tunnel: w3403 -> [_ w3509 _ w3556 _ _ _ _ _]
                  tunnel: w3399 -> [_ _ _ w3557 _ _ _ _ _]
                  tunnel: w3402 -> [_ w3508 _ _ _ _ _ _ _]
                  tunnel: w3398 -> [_ w3505 _ w3552 _ _ _ _ _]
                  frame 0, Default {
                    w3499 = 0 ("CR DEC")
                    # "Sem apontamento"
                    n2684 = call "TickTimeout.vi"() -> ("msTick"=→"TimeoutDEC 2":u32)  [unwired: 2 in, 2 out]
                    "CR DEC UTILS" <- w3499
                    "CONT DEC UTILS" <- w3499
                  }
                  frame 1 {
                    # "Envia\nComando"
                    n2685 = Subtract(x=w3506, y=w3509) -> (x-y=w3504:dbl)
                    n2686 = Absolute Value(x=w3504) -> (abs(x)=w3510:dbl)
                    n2687 = Less?(x=w3510, y=w3508) -> (x < y?=w3503:bool)
                    n2688 = case shown="False" w3503 {
                      tunnel: [w3514 3] -> w3507
                      tunnel: w3506 -> [w3513 _]
                      tunnel: w3504 -> [w3512 _]
                      tunnel: w3505 -> [w3511 _]
                      frame False {
                        # "destino"
                        # "Fora do"
